vi "StringToBool_Ctl_6b.vi"(10 "6 Bit word (str)":string) -> (1 "Bool Out":bool[](array[boolean]), 2 "Num Out":dbl[](array[numeric]), 4 "6 Bit word (str) out":string)   [LabVIEW 2018]
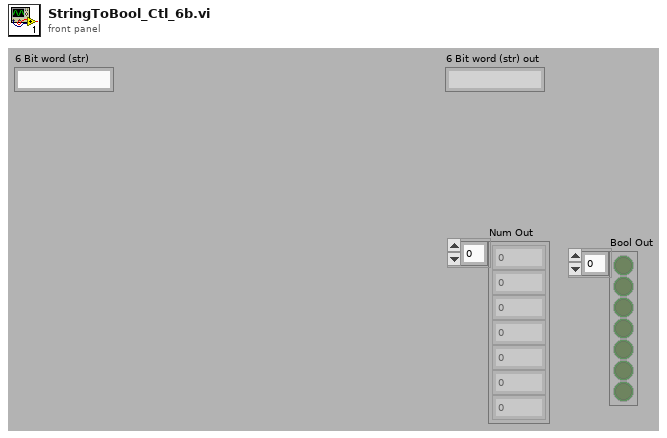
[diagram p1: front panel]
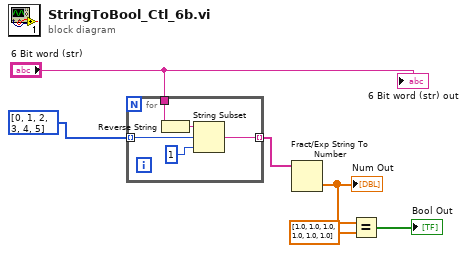
[diagram p0: block diagram]
diagram:
  n1 = for {
    tunnel: "6 Bit word (str)" -> [w11]
    tunnel: [w9] -> w4 mode=indexing
    tunnel: i32[] [0, 1, 2, 3, 4, 5] -> [w8] mode=indexing
    n2 = Reverse String(1:w11) -> (0:w7:string)
    n3 = String Subset(string=w7, offset (0)=w8, length (rest)=1 ("length (rest)")) -> (substring=w9:string)
  }
  n4 = Fract/Exp String To Number(string=w4) -> (number=w3:dbl[])  [unwired: 3 in, 1 out]
  "Num Out" <- w3
  n5 = Equal?(x=w3, y=dbl[] [1.0, 1.0, 1.0, 1.0, 1.0, 1.0]) -> (x = y?=→"Bool Out":bool[])
  "6 Bit word (str) out" <- "6 Bit word (str)"
